vi "Read Queue of Error.vi"(11 "Base Spawn in":refnum<class "Base Spawn.lvclass">) -> (2 "Queue of Error":refnum<queue>)   [LabVIEW 2025, in "jettl.lvlib" / "Spawn.lvlib" / "Base Spawn.lvclass"]
uses:
  Base Spawn.lvclass
  Base Spawn.lvclass/Base Spawn.ctl
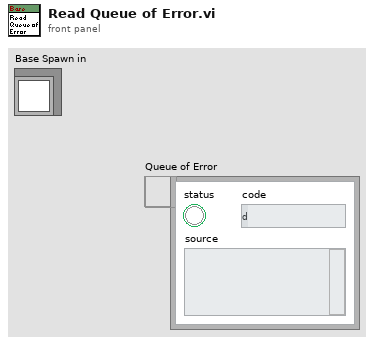
[diagram p1: front panel]
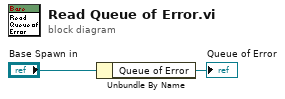
[diagram p0: block diagram]
diagram:
  n1 = Unbundle By Name("Base Spawn in") -> ("Queue of Error"=→"Queue of Error":refnum<queue>)
